vi "Register.vi"(8 "error in (no error)":errorcluster) -> (0 "error out":errorcluster, 3 "Event Registration Refnum":refnum<event-registration>)   [LabVIEW 2017, in "Log.lvclass"]
uses:
  Log.lvclass
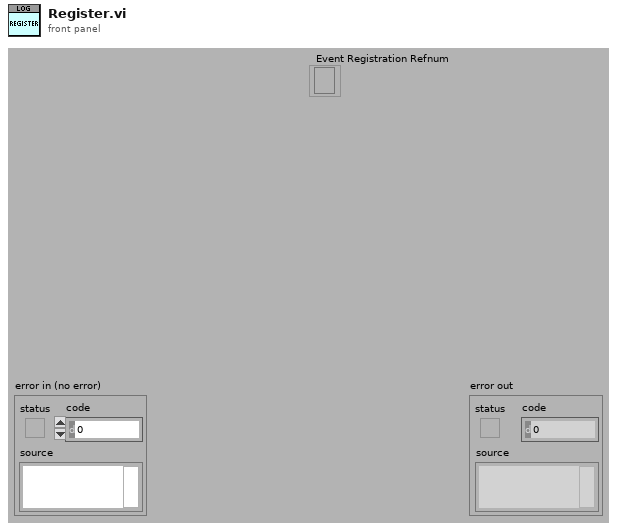
[diagram p1: front panel]
types:
  T1 = typedef "Log.lvclass/ObjectAttributes.ctl" = cluster{"Level":T2, "Facilities":variant, "Event":refnum<user-event>}
  T2 = typedef "Log.lvclass/Log_Level.ctl" = enum16{"none", "info", "trace", "warn", "error", "fatal"}
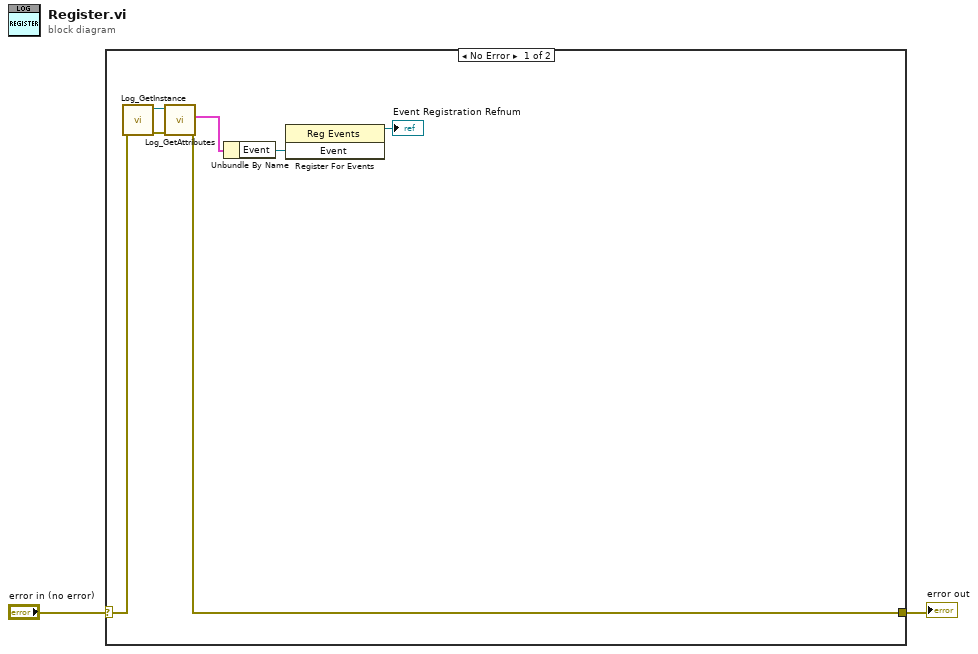
[diagram p0: block diagram]
diagram:
  n1 = case shown="No Error" "error in (no error)" {
    selector: "error in (no error)" -> [w6 w10]
    tunnel: [w8 w10] -> w1
    frame No Error {
      n2 = call "Log_GetInstance.vi"("error in (no error)"=w6) -> ("error out"=w5:errorcluster, "reference out"=w7:refnum<class "Log.lvclass">)  [unwired: 6 in, 3 out]
      n3 = call "Log_GetAttributes.vi"("error in (no error)"=w5, "reference in"=w7) -> ("error out"=w8:errorcluster, "Data"=w9:T1)  [unwired: 6 in, 2 out]
      n4 = Unbundle By Name(w9) -> ("Event"=w4:refnum<user-event>)
      n5 = register-events(w4) -> (reference out=→"Event Registration Refnum":refnum<event-registration>)  [unwired: 2 in, 1 out]
    }
    frame Error {
    }
  }
  "error out" <- w1
